vi "Lian_Lab08_II.vi"() -> ()   [LabVIEW 2020]
uses:
  <vilib>/DAQmx/read.llb/DAQmx Read (Analog 1D DBL 1Chan NSamp).vi
  <vilib>/DAQmx/create/channels.llb/DAQmx Create Channel (AI-Voltage-Basic).vi
  <vilib>/DAQmx/configure/timing.llb/DAQmx Timing (Sample Clock).vi
  <vilib>/DAQmx/miscellaneous.llb/DAQmx Fill In Error Info.vi
panel:
  out "Waveform Chart":dbl[](graph)
  in  "file path (use dialog)":path=path "C:/Users/Billy/Desktop/DAQ/Labs/Lab8/Lian_Lab08.txt"
  in  "?":bool
  in  "Loop Multiple (ms)":u32
  in  "number of samples \nper channel":i32=10
  in  "Rate":dbl=100.0 format="%0.2f"
  in  "Samples per Channel":i32=1000
  in  "Physical Channels":tag="myDAQ1/ai0"
  in  "Maximum Voltage":dbl=10.0 format="%0.2f"
  in  "Minimum Voltage":dbl=-10.0 format="%0.2f"
  in  "Input Terminal Config.":i32(ring)=10106 items=["Default"=-1, "RSE"=10083, "NRSE"=10078, "Differential"=10106, "Pseudodifferential"=12529]
  # "Part II. Saving Data to Disk"
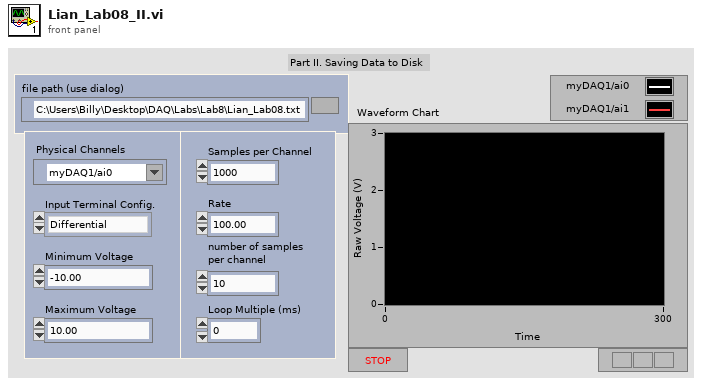
[diagram p1: front panel]
types:
  T1 = enum16{"open", "replace", "create", "open or create", "replace or create", "replace or create with confirmation"}
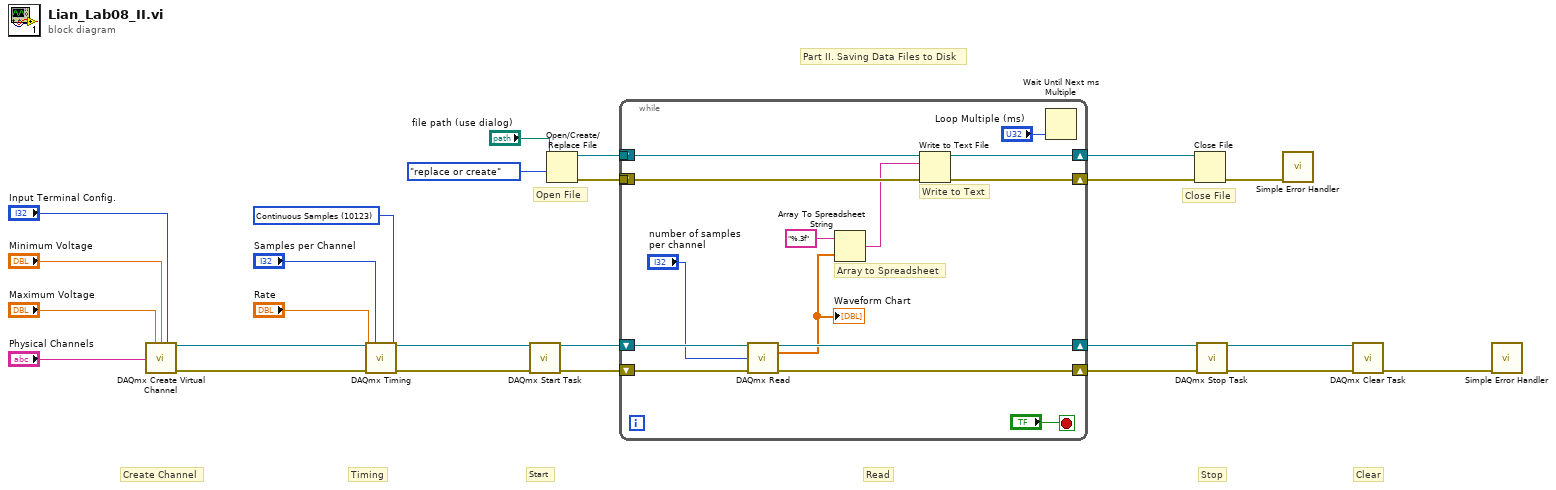
[diagram p0: block diagram]
diagram:
  w8 = 10123 items=["Finite Samples"=10178, "Continuous Samples"=10123, "Hardware Timed Single Point"=12522] ("sample mode")
  # "Close File"
  # "Open File"
  # "Part II. Saving Data Files to Disk"
  # "Clear"
  # "Stop"
  # "Read"
  # "Start"
  # "Timing"
  # "Create Channel"
  n1 = call-poly <vilib>:"DAQmx Create Virtual Channel.vi"("maximum value"="Maximum Voltage", "minimum value"="Minimum Voltage", "input terminal configuration"="Input Terminal Config.", "physical channels"="Physical Channels") -> ("task out"=w14:refnum<k21>, "error out"=w20:errorcluster)  [unwired: 10 in]
  n2 = call-poly <vilib>:"DAQmx Timing.vi"("task/channels in"=w14, "sample mode"=w8, "samples per channel"="Samples per Channel", "rate"="Rate", "error in"=w20) -> ("task out"=w13:refnum<k21>, "error out"=w19:errorcluster)  [unwired: 9 in]
  n3 = call <vilib>:"DAQmx Start Task.vi"("task/channels in"=w13, "error in"=w19) -> ("task out"=w12:refnum<k21>, "error out"=w18:errorcluster)  [unwired: 12 in]
  n4 = Open/Create/Replace File(file path (use dialog)="file path (use dialog)", operation (0:open)=T1."replace or create") -> (refnum out=w2:refnum<file>, error out=w5:errorcluster)  [unwired: 4 in, 1 out]
  n5 = while {
    shift-right: [w38] -> w17
    shift-left: w18 -> [w39]
    shift-right: [w36] -> w11
    shift-left: w12 -> [w37]
    tunnel: w5 -> [w33]
    tunnel: w2 -> [w28]
    shift-right: [w32] -> w4
    shift-left: _ -> [_]
    shift-right: [w29] -> w3
    shift-left: _ -> [_]
    stop <- "?" stop-if-true
    # "Array to Spreadsheet"
    # "Write to Text"
    n6 = call-poly <vilib>:"DAQmx Read.vi"("task/channels in"=w37, "number of samples per channel"="number of samples \nper channel", "error in"=w39) -> ("task out"=w36:refnum<k21>, "data"=w27:dbl[], "error out"=w38:errorcluster)  [unwired: 10 in]
    "Waveform Chart" <- w27
    n7 = Array To Spreadsheet String(array=w27, 3:"%.3f" ("format string")) -> (spreadsheet string=w30:string)  [unwired: 1 in]
    n8 = Write to Text File(file (use dialog)=w28, text=w30, error in=w33) -> (refnum out=w29:refnum<file>, error out=w32:errorcluster)  [unwired: 1 in, 1 out]
    n9 = Wait Until Next ms Multiple(millisecond multiple="Loop Multiple (ms)") -> ()  [unwired: 1 out]
  }
  n10 = Close File(refnum=w3, error in=w4) -> (error out=w1:errorcluster)  [unwired: 1 out]
  n11 = call <vilib>:"DAQmx Stop Task.vi"("task/channels in"=w11, "error in"=w17) -> ("task out"=w10:refnum<k21>, "error out"=w16:errorcluster)  [unwired: 12 in]
  n12 = call <vilib>:"Simple Error Handler.vi"("error in (no error)"=w1) -> ()  [unwired: 4 in, 5 out]
  n13 = call <vilib>:"DAQmx Clear Task.vi"("task in"=w10, "error in"=w16) -> ("error out"=w15:errorcluster)  [unwired: 13 in]
  n14 = call <vilib>:"Simple Error Handler.vi"("error in (no error)"=w15) -> ()  [unwired: 4 in, 5 out]
